vi "highTarget.vi"(1 "4":dbl[][](array[numeric]), 2 "3":dbl[][](array[numeric]), 3 "2":dbl[][](array[numeric]), 4 "1":dbl[][](array[numeric])) -> (0 "Highest Y":dbl[][](array[numeric]))   [LabVIEW 2011]
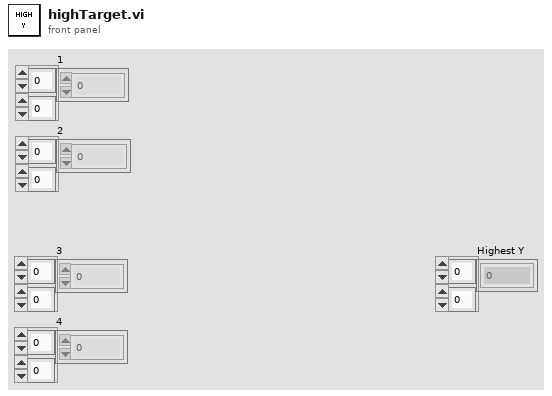
[diagram p1: front panel]
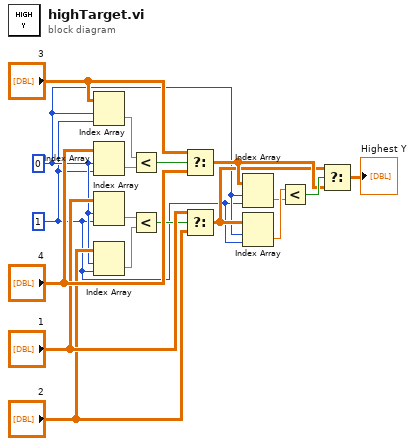
[diagram p0: block diagram]
diagram:
  w2 = 0 ("disabled index (row)")
  w1 = 1 ("disabled index (col)")
  n1 = Index Array(array="3", index (row)=w2, index (col)=w1) -> (element=w17:dbl)
  n2 = Index Array(array="4", index (row)=w2, index (col)=w1) -> (element=w16:dbl)
  n3 = Index Array(array="1", index (row)=w2, index (col)=w1) -> (element=w8:dbl)
  n4 = Index Array(array="2", index (row)=w2, index (col)=w1) -> (element=w9:dbl)
  n5 = Less?(x=w17, y=w16) -> (x < y?=w15:bool)
  n6 = Less?(x=w8, y=w9) -> (x < y?=w10:bool)
  n7 = Select(t="3", s=w15, f="4") -> (s? t:f=w4:dbl[][])
  n8 = Select(t="1", s=w10, f="2") -> (s? t:f=w3:dbl[][])
  n9 = Index Array(array=w4, index (row)=w2, index (col)=w1) -> (element=w6:dbl)
  n10 = Index Array(array=w3, index (row)=w2, index (col)=w1) -> (element=w7:dbl)
  n11 = Less?(x=w7, y=w6) -> (x < y?=w18:bool)
  n12 = Select(t=w3, s=w18, f=w4) -> (s? t:f=→"Highest Y":dbl[][])
